vi "Pigeon Status Period.vi"(8 "error in (no error)":errorcluster, 10 "Pigeon Status Config Array":T1=[{"Status Frame Enum"=270336, "STATUS_Period"=240}] {"Status Frame Enum" items=["CondStatus_1_General"=270336, "CondStatus_9_SixDeg_YPR"=270848, "CondStatus_6_SensorFusion"=270656, "CondStatus_11_GyroAccum"=270976, "CondStatus_2_GeneralCompass"=270400, "CondStatus_3_GeneralAccel"=270464, "CondStatus_10_SixDeg_Quat"=270912, "RawStatus_4_Mag"=265408, "BiasedStatus_2_Gyro"=269376, "BiasedStatus_4_Mag"=269504, "BiasedStatus_6_Accel"=269632]; "STATUS_Period" items=["Low (240ms)"=240, "Medium (50ms)"=50, "High (10ms)"=10]}, 11 "PigeonIMUDevRef":T4={"DeviceStatus"={"status"=FALSE, "code"=0, "source"=""}, "Device Number"=0, "Type"=352321536, "Device ID"=0, "Handle"=0, "UsageFrame"=0, "Library Path"=path ""} {"Type" items=["CAN"=352321536, "TalonSRX"=33554432]}) -> (0 "error out":errorcluster, 3 "PigeonIMUDevRef":T4={"DeviceStatus"={"status"=FALSE, "code"=0, "source"=""}, "Device Number"=0, "Type"=352321536, "Device ID"=0, "Handle"=0, "UsageFrame"=0, "Library Path"=path ""} {"Type" items=["CAN"=352321536, "TalonSRX"=33554432]})   [LabVIEW 2020]
uses:
  <vilib>/Rock Robotics/WPI/ThirdParty/Phoenix-LabVIEW/Pigeon IMU/CTRE_PigeonIMU_DeviceRef.ctl
  <vilib>/Rock Robotics/WPI/ThirdParty/Phoenix-LabVIEW/Pigeon IMU/CTRE_PigeonIMU_ConnectionType.ctl
  Pigeon Status Config Array.ctl
  <vilib>/Rock Robotics/WPI/ThirdParty/Phoenix-LabVIEW/Pigeon IMU/CTRE_PigeonIMU_StatusFrameRate.ctl
  STATUS_Period.ctl
  8bffcf12-d87b-4679-b93c-e69f5877cc70.vi
  <vilib>/Comparison/Equal/Equal Functor/Equal Functor.lvclass
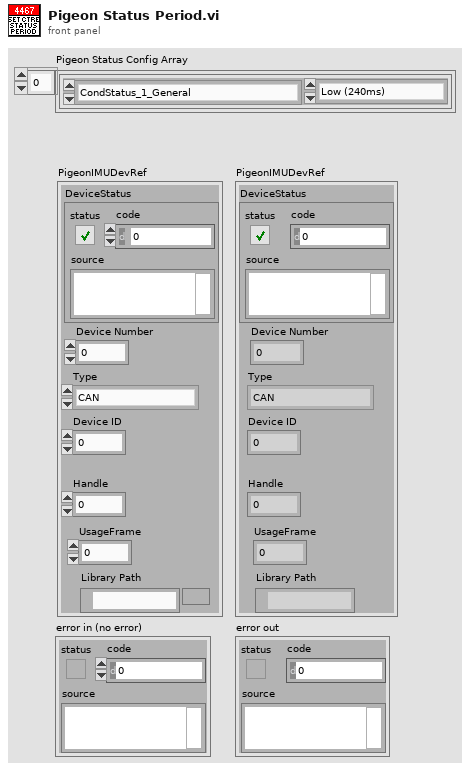
[diagram p1: front panel]
types:
  T1 = typedef "Pigeon Status Config Array.ctl" = cluster{"Status Frame Enum":T2, "STATUS_Period":T3}[]
  T2 = typedef "CTRE_PigeonIMU_StatusFrameRate.ctl" = u32
  T3 = typedef "STATUS_Period.ctl" = i32
  T4 = typedef "CTRE_PigeonIMU_DeviceRef.ctl" = cluster{"DeviceStatus":errorcluster, "Device Number":u8, "Type":T5, "Device ID":u32, "Handle":u64, "UsageFrame":u32, "Library Path":path}
  T5 = typedef "CTRE_PigeonIMU_ConnectionType.ctl" = u32
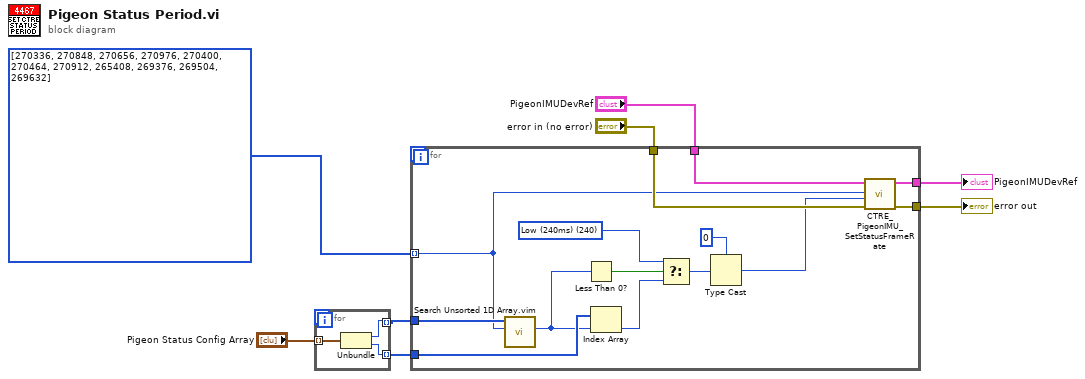
[diagram p0: block diagram]
diagram:
  w1 = T2[] [270336, 270848, 270656, 270976, 270400, 270464, 270912, 265408, 269376, 269504, 269632] items=["CondStatus_1_General"=270336, "CondStatus_9_SixDeg_YPR"=270848, "CondStatus_6_SensorFusion"=270656, "CondStatus_11_GyroAccum"=270976, "CondStatus_2_GeneralCompass"=270400, "CondStatus_3_GeneralAccel"=270464, "CondStatus_10_SixDeg_Quat"=270912, "RawStatus_4_Mag"=265408, "BiasedStatus_2_Gyro"=269376, "BiasedStatus_4_Mag"=269504, "BiasedStatus_6_Accel"=269632] ("StatusFrame")
  n1 = for {
    tunnel: "Pigeon Status Config Array" -> [w9] mode=indexing
    tunnel: [w11] -> w6 mode=indexing
    tunnel: [w10] -> w5 mode=indexing
    n2 = Unbundle(w9) -> ("Status Frame Enum"=w11:T2, "STATUS_Period"=w10:T3)
  }
  n3 = for {
    tunnel: [w25] -> w3
    tunnel: [w24] -> w8
    tunnel: w6 -> [w23]
    tunnel: w5 -> [w22]
    tunnel: "error in (no error)" -> [w18]
    tunnel: "PigeonIMUDevRef" -> [w15]
    tunnel: w1 -> [w12] mode=indexing
    w13 = T3 240 items=["Low (240ms)"=240, "Medium (50ms)"=50, "High (10ms)"=10] ("STATUS_Period")
    n4 = call "Search Unsorted 1D Array.vim"("element"=w12, "unsorted 1D array"=w23) -> ("index of element"=w21:i32)  [unwired: 9 in]
    n5 = Less Than 0?(x=w21) -> (x < 0?=w20:bool)
    n6 = Index Array(array=w22, index=w21) -> (element=w19:T3)
    n7 = Select(t=w13, s=w20, f=w19) -> (s? t:f=w17:T3)
    n8 = Type Cast(type=i16 0, x=w17) -> (*(type *) &x=w14:i16)
    n9 = call <vilib>:"CTRE_PigeonIMU_SetStatusFrameRate.vi"("error in (no error)"=w18, "Period (ms)"=w14, "StatusFrame"=w12, "PigeonIMUDevRef"=w15) -> ("error out"=w24:errorcluster, "PigeonIMUDevRef"=w25:T4)  [unwired: 6 in]
  }
  "error out" <- w8
  "PigeonIMUDevRef" <- w3
